vi "Realsense Cam Stream Profile Find.vi"(10 "Stream Config":T3={"Stream Type"=enum."Color", "Resolution"=27} {"Resolution" items=["424 x 240 @6fps", "424 x 240 @15fps", "424 x 240 @30fps", "424 x 240 @60fps", "424 x 240 @90fps", "480 x 270 @6fps", "480 x 270 @15fps", "480 x 270 @30fps", "480 x 270 @60fps", "480 x 270 @90fps", "640 x 360 @6fps", "640 x 360 @15fps", "640 x 360 @30fps", "640 x 360 @60fps", "640 x 360 @90fps", "640 x 480 @6fps", "640 x 480 @15fps", "640 x 480 @30fps", "640 x 480 @60fps", "640 x 480 @90fps", "848 x 100 @100fps", "848 x 480 @6fps", "848 x 480 @15fps", "848 x 480 @30fps", "848 x 480 @60fps", "848 x 480 @90fps", "1280 x 720 @6fps", "1280 x 720 @15fps", "1280 x 720 @30fps", "1280 x 800 @15fps", "1280 x 800 @30fps"]}, 11 "Profiles":T5) -> (3 "Stream":T1)   [LabVIEW 2018, in "Realsense Cam.lvclass"]
uses:
  Realsense Cam.lvclass
  Private/Cam Profiles STYP.ctl
  Private/Stream STYP.ctl
  Private/Stream Frame Data STYP.ctl
  Private/Stream Config STYP.ctl
  Private/Stream Types Enum STYP.ctl
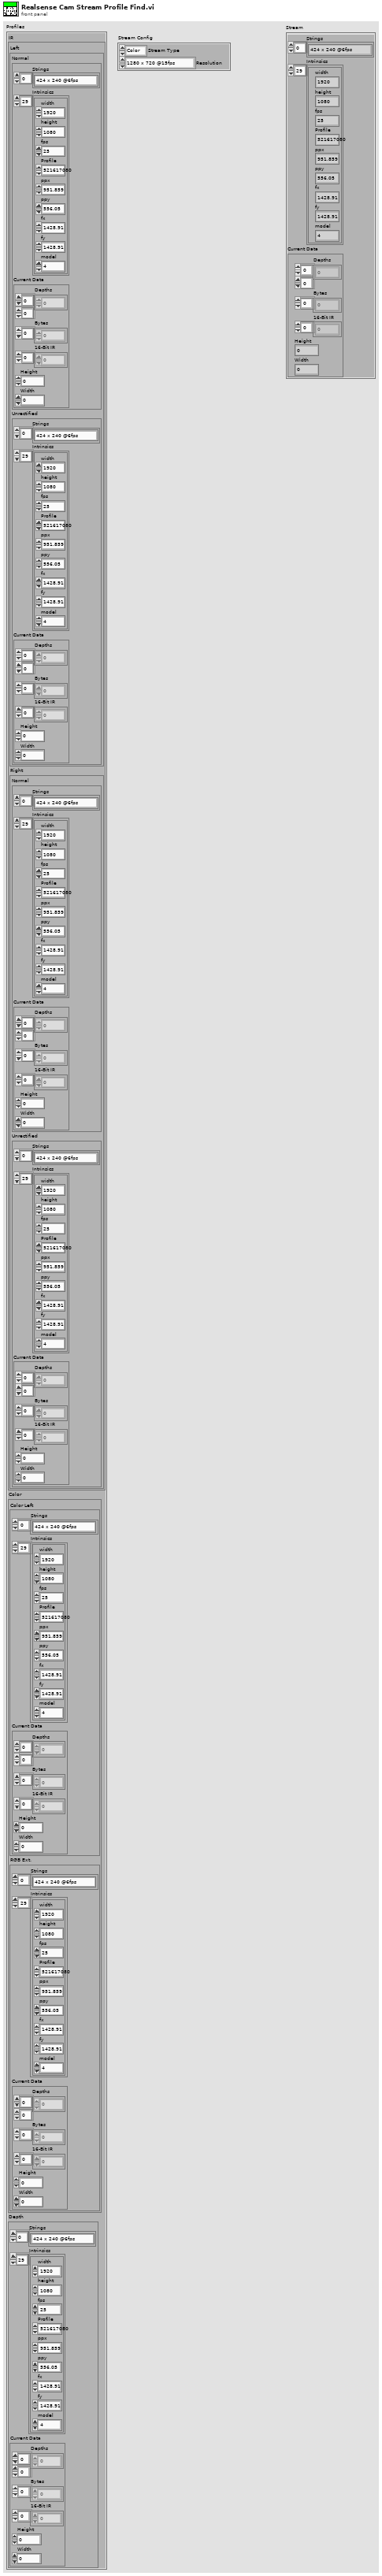
[diagram p1: front panel]
types:
  T1 = typedef "Realsense Cam.lvclass/Stream STYP.ctl" = cluster{"Strings":string[], "Intrinsics":cluster{"width":i32, "height":i32, "fps":i32, "Profile":u64, "ppx":sgl, "ppy":sgl, "fx":sgl, "fy":sgl, "model":u32}[], "Current Data":T2}
  T2 = typedef "Realsense Cam.lvclass/Stream Frame Data STYP.ctl" = cluster{"Depths":sgl[][], "Bytes":u8[], "16-Bit IR":u16[], "Height":i32, "Width":i32}
  T3 = typedef "Realsense Cam.lvclass/Stream Config STYP.ctl" = cluster{"Stream Type":T4, "Resolution":u16}
  T4 = typedef "Realsense Cam.lvclass/Stream Types Enum STYP.ctl" = enum16{"Depth", "Left IR", "Left IR Unrectified", "Right IR", "Right IR Unrectified", "Color", "RGB Ext."}
  T5 = typedef "Realsense Cam.lvclass/Cam Profiles STYP.ctl" = cluster{"IR":cluster{"Left":cluster{"Normal":T1, "Unrectified":T1}, "Right":cluster{"Normal":T1, "Unrectified":T1}}, "Color":cluster{"Color Left":T1, "RGB Ext.":T1}, "Depth":T1}
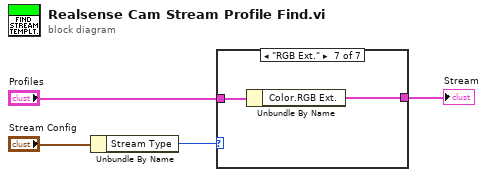
[diagram p0: block diagram]
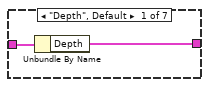
[diagram p2: hidden frame]
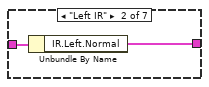
[diagram p3: hidden frame]
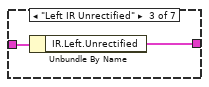
[diagram p4: hidden frame]
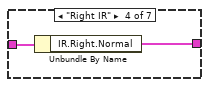
[diagram p5: hidden frame]
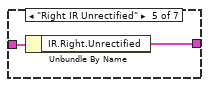
[diagram p6: hidden frame]
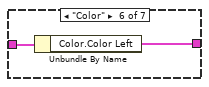
[diagram p7: hidden frame]
diagram:
  n1 = Unbundle By Name("Stream Config") -> ("Stream Type"=w3:T4)
  n2 = case shown="\"RGB Ext.\"" w3 {
    tunnel: "Profiles" -> [w6 w8 w10 w12 w14 w16 w18]
    tunnel: [w5 w7 w9 w11 w13 w15 w17] -> w1
    frame "Depth", Default {
      n3 = Unbundle By Name(w6) -> ("Depth"=w5:T1)
    }
    frame "Left IR" {
      n4 = Unbundle By Name(w8) -> ("IR.Left.Normal"=w7:T1)
    }
    frame "Left IR Unrectified" {
      n5 = Unbundle By Name(w10) -> ("IR.Left.Unrectified"=w9:T1)
    }
    frame "Right IR" {
      n6 = Unbundle By Name(w12) -> ("IR.Right.Normal"=w11:T1)
    }
    frame "Right IR Unrectified" {
      n7 = Unbundle By Name(w14) -> ("IR.Right.Unrectified"=w13:T1)
    }
    frame "Color" {
      n8 = Unbundle By Name(w16) -> ("Color.Color Left"=w15:T1)
    }
    frame "RGB Ext." {
      n9 = Unbundle By Name(w18) -> ("Color.RGB Ext."=w17:T1)
    }
  }
  "Stream" <- w1
